vi "LabVIEW 1.vi"() -> ()   [LabVIEW 2020]
panel:
  out "Numérique":i32
  out "Indicateur Chaîne":string
  out "Indicateur Booléen":bool
  in  "Commande Booléen":bool
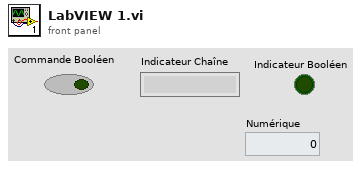
[diagram p1: front panel]
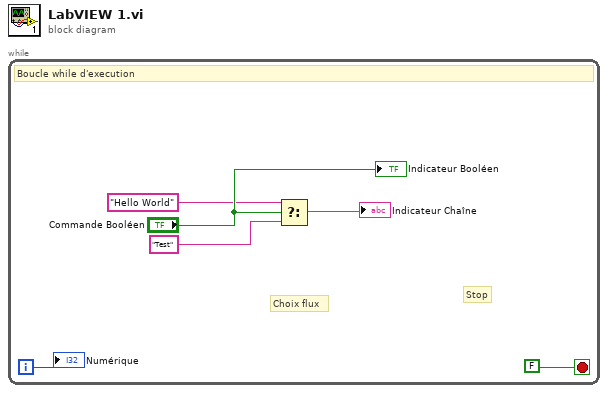
[diagram p0: block diagram]
diagram:
  n1 = while {
    i -> [w1]
    stop <- FALSE stop-if-true
    # "Choix flux"
    # "Stop"
    # "Boucle while d'execution"
    n2 = Select(t="Hello World" ("Commande Chaîne"), s="Commande Booléen", f="Test") -> (s? t:f=→"Indicateur Chaîne":string)
    "Indicateur Booléen" <- "Commande Booléen"
    "Numérique" <- w1
  }
